vi "Robot Global Data.vi"() -> ()   [LabVIEW 2014]
doc: "This global VI can contain as many global variables as you need. Place a control on the panel, give it a good name. To read or write to it from a VI, drag the icon to the diagram of that VI. You can also drag from the project. Click on the node to change which global you access. You shouldn't have multiple locations writing to a global or it will cause a race-condition."
uses:
  <vilib>/Rock Robotics/WPI/Camera/WPI_CameraImageSize.ctl
  <vilib>/Rock Robotics/WPI/DriverStation/WPI_DriverStationRobotMode2.ctl
  <vilib>/Rock Robotics/SystemInterfaces/DIO/FPGA_DIOChannel.ctl
panel:
  in  "Motor Safety Timeout":dbl=1.0
  in  "Wheel Difference":dbl=1.33
  out "Input Values":T1
  out "CAN and DIO IDs":T3
  in  "Robot Mode":T4
  in  "image size":T5=enum."320x240"
  in  "Enable Vision":bool
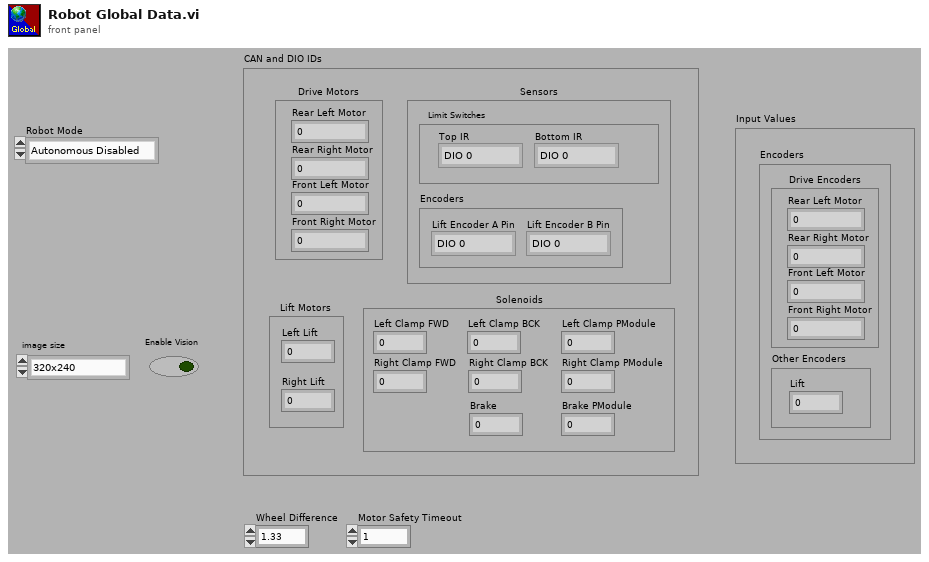
[diagram p1: front panel]
types:
  T1 = cluster{"Encoders":cluster{"Drive Encoders":cluster{"Rear Left Motor":dbl, "Rear Right Motor":dbl, "Front Left Motor":dbl, "Front Right Motor":dbl}, "Other Encoders":cluster{"Lift":dbl}}}
  T2 = typedef "FPGA_DIOChannel.ctl" = enum8{"DIO 0", "DIO 1", "DIO 2", "DIO 3", "DIO 4", "DIO 5", "DIO 6", "DIO 7", "DIO 8", "DIO 9", "DIO MXP 0", "DIO MXP 1", "DIO MXP 2", "DIO MXP 3", "DIO MXP 4", "DIO MXP 5", "DIO MXP 6", "DIO MXP 7", "DIO MXP 8", "DIO MXP 9", "DIO MXP 10", "DIO MXP 11", "DIO MXP 12", "DIO MXP 13", "DIO MXP 14", "DIO MXP 15", "Invalid"}
  T3 = cluster{"Lift Motors":cluster{"Left Lift":dbl, "Right Lift":dbl}, "Sensors":cluster{"Limit Switches":cluster{"Bottom IR":T2, "Top IR":T2}, "Encoders":cluster{"Lift Encoder A Pin":T2, "Lift Encoder B Pin":T2}}, "Solenoids":cluster{"Left Clamp FWD":dbl, "Right Clamp FWD":dbl, "Brake":dbl, "Left Clamp BCK":dbl, "Right Clamp BCK":dbl, "Left Clamp PModule":dbl, "Right Clamp PModule":dbl, "Brake PModule":dbl}, "Drive Motors":cluster{"Rear Left Motor":dbl, "Rear Right Motor":dbl, "Front Left Motor":dbl, "Front Right Motor":dbl}}
  T4 = typedef "WPI_DriverStationRobotMode2.ctl" = enum16{"Autonomous Disabled", "Autonomous Enabled", "Teleop Disabled", "Teleop Enabled", "Disconnected", "Finish", "Test Disabled", "Test Enabled", "Emergency Stopped"}
  T5 = typedef "WPI_CameraImageSize.ctl" = enum16{"640x480", "320x240", "160x120", "Custom"}
diagram:
